vi "Einstellungen Diagramme.vi"() -> ()   [LabVIEW 2020, in "Grafik.lvlib"]
uses:
  Grafik.lvlib
  Visualisierungs Elemente/Button.ctl
  Visualisierungs Elemente/Zahlen-Eingabefeld.ctl
  Visualisierungs Elemente/Auswahlfeld.ctl
  Aktionen Konfig Diagramme.ctl
  Allgemein/allgemeine Sub-VIs.lvlib
panel:
  in  "Auto Scale 6":bool
  in  "Auto Scale 5":bool
  in  "Auto Scale 4":bool
  in  "Auto Scale 3":bool
  in  "Auto Scale 2":bool
  in  "Auto Scale 1":bool
  in  "Mittelwertanzeige":bool
  in  "Werte":i32=2 min=2 max=200 step=1
  in  "X Anzeigedauer":T1 items=["5 min"=3000, "10 min"=6000, "15 min"=9000, "20 min"=12000, "30 min"=18000, "45 min"=27000, "1 h"=36000, "1,5 h"=54000]
  in  "Y Anzeige MAX":T3 {"Y Anzeige MAX 6" format="%#_5g"; "Y Anzeige MAX 5" format="%#_5g"; "Y Anzeige MAX 4" format="%#_5g"; "Y Anzeige MAX 3" format="%#_5g"; "Y Anzeige MAX 2" format="%#_5g"; "Y Anzeige MAX 1" format="%#_5g"}
  in  "Y Anzeige MIN":T4 {"Y Anzeige MIN 6" format="%#_5g"; "Y Anzeige MIN 5" format="%#_5g"; "Y Anzeige MIN 4" format="%#_5g"; "Y Anzeige MIN 3" format="%#_5g"; "Y Anzeige MIN 2" format="%#_5g"; "Y Anzeige MIN 1" format="%#_5g"}
  in  "Auto Scale X":bool
  in  "Auto Scale Y":bool
  in  "Stopp":T5
  # "Konfiguration Grafik"
  # "Anzeigedauer X-Achse:"
  # "Auto-Skalierung X:"
  # "Y Anzeige MIN:"
  # "Y Anzeige MAX:"
  # "Skalieren\naktiv:"
  # "Graph 1:"
  # "Graph 2:"
  # "Graph 3:"
  # "Graph 4:"
  # "Graph 5:"
  # "Graph 6:"
  # "Auto-Skalierung Y:"
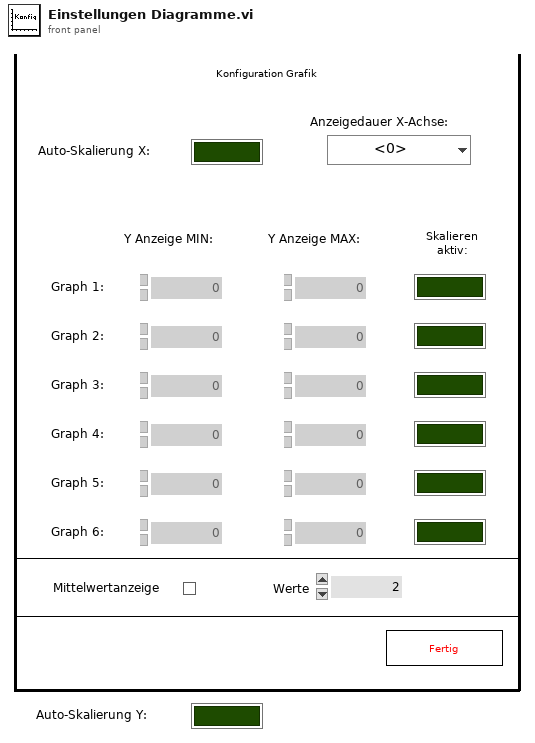
[diagram p1: front panel]
types:
  T1 = typedef "Auswahlfeld.ctl" = u16
  T2 = typedef "Zahlen-Eingabefeld.ctl" = sgl
  T3 = cluster{"Y Anzeige MAX 1":T2, "Y Anzeige MAX 2":T2, "Y Anzeige MAX 3":T2, "Y Anzeige MAX 4":T2, "Y Anzeige MAX 5":T2, "Y Anzeige MAX 6":T2}
  T4 = cluster{"Y Anzeige MIN 1":T2, "Y Anzeige MIN 2":T2, "Y Anzeige MIN 3":T2, "Y Anzeige MIN 4":T2, "Y Anzeige MIN 5":T2, "Y Anzeige MIN 6":T2}
  T5 = typedef "Button.ctl" = bool
  T6 = typedef "Grafik.lvlib/Aktionen Konfig Diagramme.ctl" = enum16{"lesen", "laden", "speichern", "X Auto Scale", "Y Auto Scale", "Anzeigedauer", "Y MIN", "Y MAX", "Referenzen", "Werteanzahl", "Autoscale einzeln"}
  T7 = enum8{"Enabled", "Disabled", "Disabled and Grayed Out"}
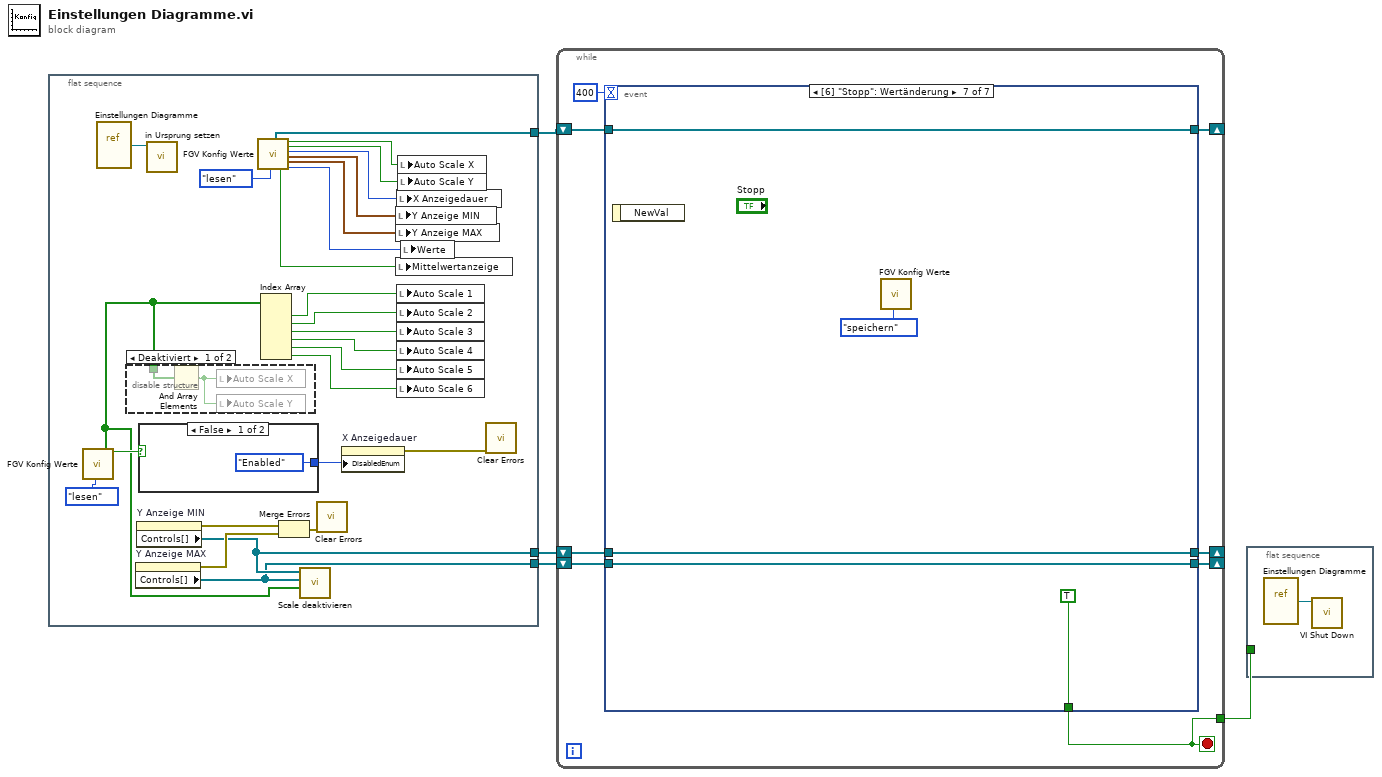
[diagram p0: block diagram]
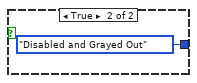
[diagram p3: hidden frame]
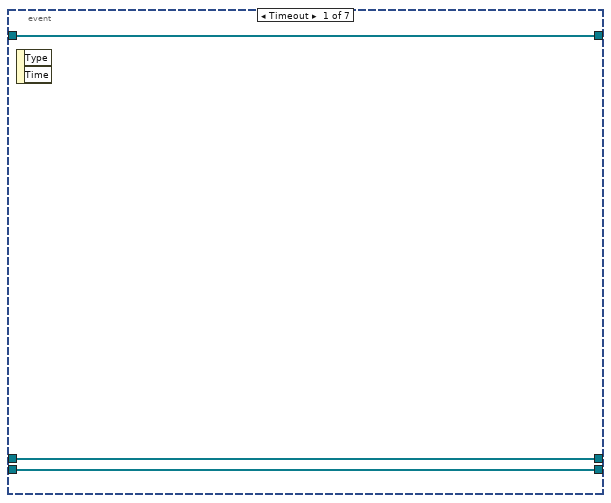
[diagram p4: hidden frame]
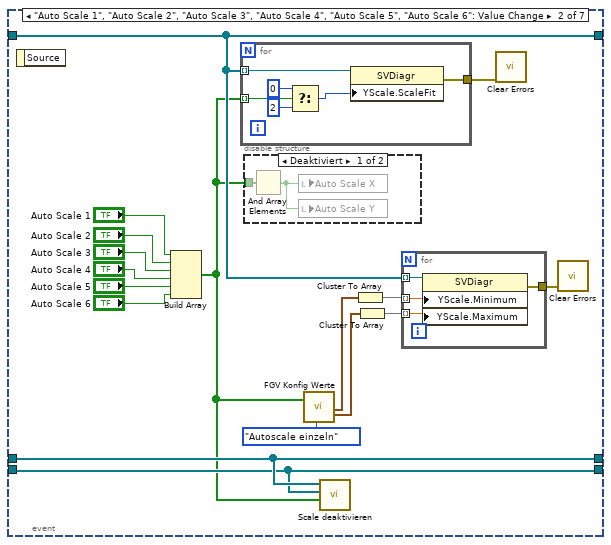
[diagram p5: hidden frame]
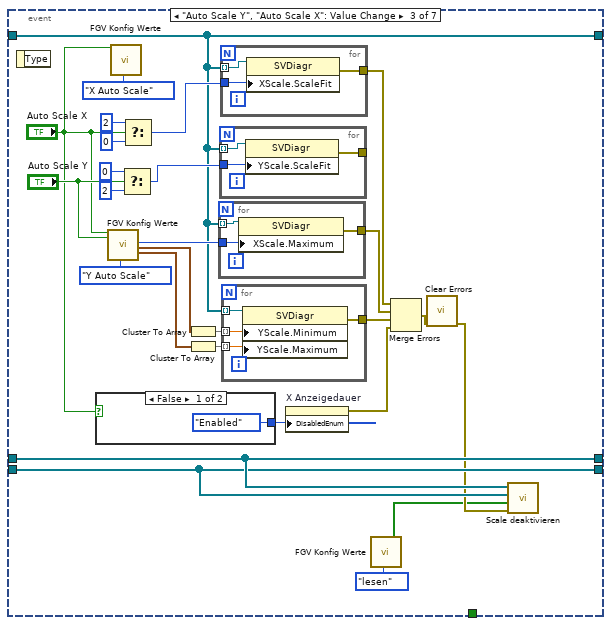
[diagram p7: hidden frame]
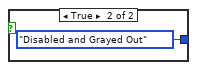
[diagram p8: hidden frame]
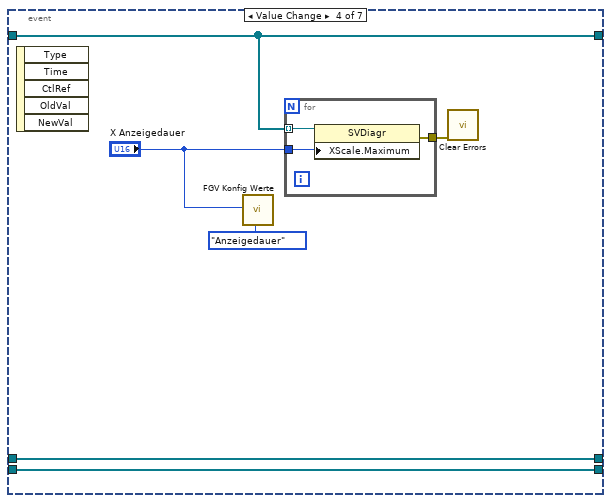
[diagram p9: hidden frame]
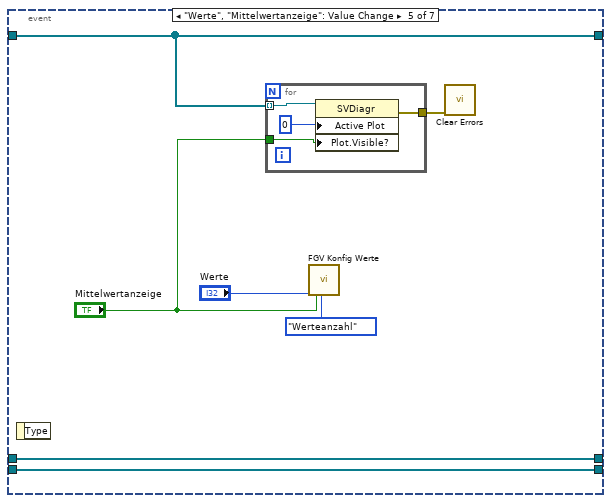
[diagram p10: hidden frame]
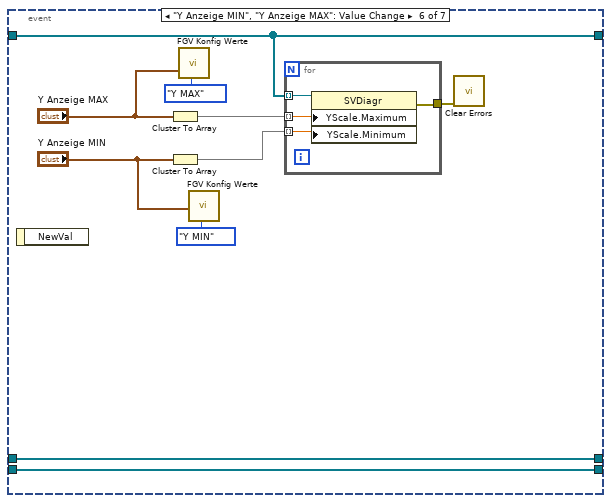
[diagram p11: hidden frame]
diagram:
  n1 = flat-sequence {
    tunnel: [w29] -> w3
    tunnel: [w14] -> w2
    tunnel: [w13] -> w1
    frame #0 {
      n2 = call "FGV Konfig Werte.vi"("Aktionen"=Aktionen_Konfig_Diagramme."lesen" ("Aktionen Konfig Diagramme")) -> ("Autoscale einzeln"=w5:bool[], "Auto Scale X"=w6:bool)  [unwired: 10 in, 7 out]
      n3 = vi-ref "Einstellungen Diagramme.vi"() -> (w19:refnum<vi>)
      n4 = disable-structure shown="Deaktiviert" {
        disable-tunnel: w5 -> [w31 _]
        frame Disabled {
          n5 = And Array Elements(Boolean array=w31) -> (logical AND=w32:bool)
          n6 = local write "Auto Scale X"(w32) -> ()
          n7 = local write "Auto Scale Y"(w32) -> ()
        }
        frame Enabled {
        }
      }
      n8 = property on="Y Anzeige MAX" class="Cluster (strikt)"() -> (error out=w17:errorcluster, "Controls[]"=w13:refnum<vi>[])  [unwired: 2 in, 1 out]
      n9 = property on="Y Anzeige MIN" class="Cluster (strikt)"() -> (error out=w15:errorcluster, "Controls[]"=w14:refnum<vi>[])  [unwired: 2 in, 1 out]
      n10 = case shown="False" w6 {
        tunnel: [T7."Enabled" ("Deaktiviert") T7."Disabled and Grayed Out" ("Deaktiviert")] -> w22
        frame False {
        }
        frame True {
        }
      }
      n11 = call "in Ursprung setzen.vi"("VI Referenz"=w19) -> ()  [unwired: 10 in, 1 out]
      n12 = call "FGV Konfig Werte.vi"("Aktionen"=Aktionen_Konfig_Diagramme."lesen" ("Aktionen Konfig Diagramme")) -> ("Referenzen"=w29:refnum<vi>[], "Mittelwertanzeige"=w20:bool, "Auto Scale X"=w28:bool, "Auto Scale Y"=w27:bool, "X Anzeigedauer"=w26:T1, "Y Anzeige MIN"=w25:T4, "Y Anzeige MAX"=w24:T3, "Werteanzeige"=w21:i32)  [unwired: 10 in, 1 out]
      n13 = Index Array(array=w5) -> (element #1=w12:bool, element #2=w11:bool, element #3=w10:bool, element #4=w9:bool, element #5=w8:bool, element #6=w7:bool)  [unwired: 6 in]
      n14 = Merge Errors(w15, w17) -> (w16:errorcluster)
      n15 = call "Scale deaktivieren.vi"("Autoscale einzeln"=w5, "Y Anzeige MAX"=w13, "Y Anzeige MIN"=w14) -> ()  [unwired: 8 in, 1 out]
      n16 = call <vilib>:"Clear Errors.vi"("error in (no error)"=w16) -> ()  [unwired: 5 in, 2 out]
      n17 = property on="X Anzeigedauer" class="Ring (strikt)"("DisabledEnum"=w22) -> (error out=w18:errorcluster)  [unwired: 2 in, 1 out]
      n18 = local write "Y Anzeige MIN"(w25) -> ()
      n19 = local write "Y Anzeige MAX"(w24) -> ()
      n20 = local write "Mittelwertanzeige"(w20) -> ()
      n21 = local write "X Anzeigedauer"(w26) -> ()
      n22 = local write "Auto Scale 1"(w12) -> ()
      n23 = local write "Auto Scale 2"(w11) -> ()
      n24 = local write "Auto Scale 3"(w10) -> ()
      n25 = local write "Auto Scale 4"(w9) -> ()
      n26 = local write "Auto Scale 5"(w8) -> ()
      n27 = local write "Auto Scale 6"(w7) -> ()
      n28 = local write "Auto Scale X"(w28) -> ()
      n29 = local write "Auto Scale Y"(w27) -> ()
      n30 = local write "Werte"(w21) -> ()
      n31 = call <vilib>:"Clear Errors.vi"("error in (no error)"=w18) -> ()  [unwired: 5 in, 2 out]
    }
  }
  n32 = while {
    tunnel: [w41] -> w4
    shift-right: [w36] -> _
    shift-left: w1 -> [w37]
    shift-right: [w39] -> _
    shift-left: w2 -> [w38]
    shift-right: [w35] -> _
    shift-left: w3 -> [w40]
    stop <- w41 stop-if-true
    n33 = event shown="[6] \"Stopp\": Wertänderung" {
      selector: _ -> [_ _ _ _ _ _ _]
      dyn-events: _ -> [_ _ _ _ _ _ _]
      timeout: 400 -> [_ _ _ _ _ _ _]
      tunnel: [_ _ _ _ _ _ TRUE] -> w41
      tunnel: w40 -> [w43 w52 w80 w117 w126 w137 w152]
      tunnel: [w45 w55 w85 w119 w128 w139 w154] -> w39
      tunnel: w38 -> [w45 w55 w85 w119 w128 w139 w154]
      tunnel: [w44 w54 w84 w118 w127 w138 w153] -> w36
      tunnel: w37 -> [w44 w54 w84 w118 w127 w138 w153]
      tunnel: [w43 w52 w80 w117 w126 w137 w152] -> w35
      event Timeout {
        n34 = event-data() -> ()  [unwired: 1 in, 2 out]
      }
      event "Auto Scale 1", "Auto Scale 2", "Auto Scale 3", "Auto Scale 4", "Auto Scale 5", "Auto Scale 6": Value Change {
        n35 = event-data() -> ()  [unwired: 1 in, 1 out]
        n36 = Build Array("Auto Scale 1", "Auto Scale 2", "Auto Scale 3", "Auto Scale 4", "Auto Scale 5", "Auto Scale 6") -> (w46:bool[])
        n37 = for {
          tunnel: [w74] -> w53
          tunnel: w52 -> [w73] mode=indexing
          tunnel: w46 -> [w70] mode=indexing
          n38 = Select(t=u8 0 ("X-Achse.Achsenanpassung"), s=w70, f=u8 2 ("X-Achse.Achsenanpassung")) -> (s? t:f=w69:u8)
          n39 = property on="Eigenschaftsknoten" class="SVDiagr"(reference=w73, "YScale.ScaleFit"=w69) -> (error out=w74:errorcluster)  [unwired: 1 in, 1 out]
        }
        n40 = disable-structure shown="Deaktiviert" {
          disable-tunnel: w46 -> [w64 _]
          frame Disabled {
            n41 = And Array Elements(Boolean array=w64) -> (logical AND=w63:bool)
            n42 = local write "Auto Scale X"(w63) -> ()
            n43 = local write "Auto Scale Y"(w63) -> ()
          }
          frame Enabled {
          }
        }
        n44 = call "FGV Konfig Werte.vi"("Autoscale einzeln"=w46, "Aktionen"=Aktionen_Konfig_Diagramme."Autoscale einzeln") -> ("Y Anzeige MIN"=w51:T4, "Y Anzeige MAX"=w49:T3)  [unwired: 9 in, 7 out]
        n45 = call "Scale deaktivieren.vi"("Autoscale einzeln"=w46, "Y Anzeige MAX"=w54, "Y Anzeige MIN"=w55) -> ()  [unwired: 8 in, 1 out]
        n46 = Cluster To Array(cluster=w51) -> (array=w50:T2[])
        n47 = Cluster To Array(cluster=w49) -> (array=w48:T2[])
        n48 = for {
          tunnel: w50 -> [w68] mode=indexing
          tunnel: w48 -> [w67] mode=indexing
          tunnel: w52 -> [w66] mode=indexing
          tunnel: [w65] -> w47
          n49 = property on="Eigenschaftsknoten" class="SVDiagr"(reference=w66, "YScale.Minimum"=w68, "YScale.Maximum"=w67) -> (error out=w65:errorcluster)  [unwired: 1 in, 1 out]
        }
        n50 = call <vilib>:"Clear Errors.vi"("error in (no error)"=w53) -> ()  [unwired: 5 in, 2 out]
        n51 = call <vilib>:"Clear Errors.vi"("error in (no error)"=w47) -> ()  [unwired: 5 in, 2 out]
      }
      event "Auto Scale Y", "Auto Scale X": Value Change {
        n52 = event-data() -> ()  [unwired: 1 in, 1 out]
        n53 = case shown="False" "Auto Scale X" {
          tunnel: [T7."Enabled" ("Deaktiviert") T7."Disabled and Grayed Out" ("Deaktiviert")] -> w91
          frame False {
          }
          frame True {
          }
        }
        n54 = call "FGV Konfig Werte.vi"("Auto Scale X"="Auto Scale X", "Auto Scale Y"="Auto Scale Y", "Aktionen"=Aktionen_Konfig_Diagramme."Y Auto Scale" ("Aktionen Konfig Diagramme")) -> ("X Anzeigedauer"=w96:T1, "Y Anzeige MIN"=w94:T4, "Y Anzeige MAX"=w95:T3)  [unwired: 8 in, 6 out]
        n55 = call "FGV Konfig Werte.vi"("Auto Scale X"="Auto Scale X", "Aktionen"=Aktionen_Konfig_Diagramme."X Auto Scale" ("Aktionen Konfig Diagramme")) -> ()  [unwired: 9 in, 9 out]
        n56 = Select(t=u8 0 ("X-Achse.Achsenanpassung"), s="Auto Scale Y", f=u8 2 ("X-Achse.Achsenanpassung")) -> (s? t:f=w81:u8)
        n57 = Select(t=u8 2 ("X-Achse.Achsenanpassung"), s="Auto Scale X", f=u8 0 ("X-Achse.Achsenanpassung")) -> (s? t:f=w99:u8)
        n58 = Cluster To Array(cluster=w94) -> (array=w93:T2[])
        n59 = Cluster To Array(cluster=w95) -> (array=w92:T2[])
        n60 = for {
          tunnel: w96 -> [w109]
          tunnel: w80 -> [w108] mode=indexing
          tunnel: [w107] -> w88
          n61 = property on="Eigenschaftsknoten" class="SVDiagr"(reference=w108, "XScale.Maximum"=w109) -> (error out=w107:errorcluster)  [unwired: 1 in, 1 out]
        }
        n62 = for {
          tunnel: w80 -> [w104] mode=indexing
          tunnel: w81 -> [w103]
          tunnel: [w102] -> _
          n63 = property on="Eigenschaftsknoten" class="SVDiagr"(reference=w104, "YScale.ScaleFit"=w103) -> (error out=w102:errorcluster)  [unwired: 1 in, 1 out]
        }
        n64 = for {
          tunnel: w80 -> [w116] mode=indexing
          tunnel: w99 -> [w115]
          tunnel: [w114] -> w87
          n65 = property on="Eigenschaftsknoten" class="SVDiagr"(reference=w116, "XScale.ScaleFit"=w115) -> (error out=w114:errorcluster)  [unwired: 1 in, 1 out]
        }
        n66 = for {
          tunnel: w93 -> [w113] mode=indexing
          tunnel: w92 -> [w112] mode=indexing
          tunnel: w80 -> [w111] mode=indexing
          tunnel: [w110] -> w90
          n67 = property on="Eigenschaftsknoten" class="SVDiagr"(reference=w111, "YScale.Minimum"=w113, "YScale.Maximum"=w112) -> (error out=w110:errorcluster)  [unwired: 1 in, 1 out]
        }
        n68 = property on="X Anzeigedauer" class="Ring (strikt)"("DisabledEnum"=w91) -> (error out=w89:errorcluster)  [unwired: 2 in, 1 out]
        n69 = call "FGV Konfig Werte.vi"("Aktionen"=Aktionen_Konfig_Diagramme."lesen") -> ("Autoscale einzeln"=w75:bool[])  [unwired: 10 in, 8 out]
        n70 = Merge Errors(w87, w88, w90, w89) -> (w86:errorcluster)
        n71 = call <vilib>:"Clear Errors.vi"("error in (no error)"=w86) -> ("error out"=w77:errorcluster)  [unwired: 5 in, 1 out]
        n72 = call "Scale deaktivieren.vi"("error in (no error)"=w77, "Autoscale einzeln"=w75, "Y Anzeige MAX"=w84, "Y Anzeige MIN"=w85) -> ()  [unwired: 7 in, 1 out]
      }
      event Value Change {
        n73 = event-data() -> ()  [unwired: 1 in, 5 out]
        n74 = call "FGV Konfig Werte.vi"("X Anzeigedauer"="X Anzeigedauer", "Aktionen"=Aktionen_Konfig_Diagramme."Anzeigedauer" ("Aktionen Konfig Diagramme")) -> ()  [unwired: 9 in, 9 out]
        n75 = for {
          tunnel: "X Anzeigedauer" -> [w125]
          tunnel: w117 -> [w124] mode=indexing
          tunnel: [w123] -> w120
          n76 = property on="Eigenschaftsknoten" class="SVDiagr"(reference=w124, "XScale.Maximum"=w125) -> (error out=w123:errorcluster)  [unwired: 1 in, 1 out]
        }
        n77 = call <vilib>:"Clear Errors.vi"("error in (no error)"=w120) -> ()  [unwired: 5 in, 2 out]
      }
      event "Werte", "Mittelwertanzeige": Value Change {
        n78 = event-data() -> ()  [unwired: 1 in, 1 out]
        n79 = for {
          tunnel: w126 -> [w136] mode=indexing
          tunnel: "Mittelwertanzeige" -> [w134]
          tunnel: [w133] -> w129
          n80 = property class="SVDiagr"(reference=w136, "Active Plot"=u32 0 ("Aktiver Plot"), "Plot.Visible?"=w134) -> (error out=w133:errorcluster)  [unwired: 1 in, 1 out]
        }
        n81 = call "FGV Konfig Werte.vi"("Werteanzeige"="Werte", "Mittelwertanzeige"="Mittelwertanzeige", "Aktionen"=Aktionen_Konfig_Diagramme."Werteanzahl" ("Aktionen Konfig Diagramme")) -> ()  [unwired: 8 in, 9 out]
        n82 = call <vilib>:"Clear Errors.vi"("error in (no error)"=w129) -> ()  [unwired: 5 in, 2 out]
      }
      event "Y Anzeige MIN", "Y Anzeige MAX": Value Change {
        n83 = event-data() -> ()  [unwired: 1 in, 1 out]
        n84 = Cluster To Array(cluster="Y Anzeige MAX") -> (array=w146:T2[])
        n85 = Cluster To Array(cluster="Y Anzeige MIN") -> (array=w145:T2[])
        n86 = call "FGV Konfig Werte.vi"("Y Anzeige MAX"="Y Anzeige MAX", "Aktionen"=Aktionen_Konfig_Diagramme."Y MAX" ("Aktionen Konfig Diagramme")) -> ()  [unwired: 9 in, 9 out]
        n87 = call "FGV Konfig Werte.vi"("Y Anzeige MIN"="Y Anzeige MIN", "Aktionen"=Aktionen_Konfig_Diagramme."Y MIN" ("Aktionen Konfig Diagramme")) -> ()  [unwired: 9 in, 9 out]
        n88 = for {
          tunnel: w146 -> [w150] mode=indexing
          tunnel: w145 -> [w149] mode=indexing
          tunnel: w137 -> [w148] mode=indexing
          tunnel: [w147] -> w140
          n89 = property on="Eigenschaftsknoten" class="SVDiagr"(reference=w148, "YScale.Maximum"=w150, "YScale.Minimum"=w149) -> (error out=w147:errorcluster)  [unwired: 1 in, 1 out]
        }
        n90 = call <vilib>:"Clear Errors.vi"("error in (no error)"=w140) -> ()  [unwired: 5 in, 2 out]
      }
      event Value Change {
        n91 = event-data() -> ()  [unwired: 1 in, 1 out]
        n92 = call "FGV Konfig Werte.vi"("Aktionen"=Aktionen_Konfig_Diagramme."speichern" ("Aktionen Konfig Diagramme")) -> ()  [unwired: 10 in, 9 out]
      }
    }
  }
  n93 = flat-sequence {
    tunnel: w4 -> [_]
    frame #0 {
      n94 = vi-ref "Einstellungen Diagramme.vi"() -> (w156:refnum<vi>)
      n95 = call "VI Shut Down.vi"("VI Referenz"=w156) -> ()  [unwired: 11 in]
    }
  }
